vi "Simulation Trace Element.vi"(8 "error in (no error)":errorcluster, 10 "sensors":T5={"net distance (mm)"=0, "net angle (deg)"=0, "accelerometer"={"x axis (g)"=0.0, "y axis (g)"=0.0, "z axis (g)"=0.0}, "iRobot Sensors"={"Bumps + Wheel Drops"={"Wheeldrop Caster"=FALSE, "Wheeldrop Left"=FALSE, "Wheeldrop Right"=FALSE, "Bump Left"=FALSE, "Bump Right"=FALSE}, "Wall"=FALSE, "Cliff Left"=FALSE, "Cliff Front Left"=FALSE, "Cliff Front Right"=FALSE, "Cliff Right"=FALSE, "Wall Signal"=0, "Cliff Left Signal"=0, "Cliff Front Left Signal"=0, "Cliff Front Right Signal"=0, "Cliff Right Signal"=0, "Buttons"={"Advance"=FALSE, "Play"=FALSE}, "Virtual Wall"=FALSE, "# Stream Packets"=0, "Requested Velocity (mm/s)"=0, "Requested Radius (mm)"=0, "Requested Right Wheel Velocity (mm/s)"=0, "Requested Left Wheel Velocity (mm/s)"=0, "Distance (mm)"=0, "Angle (deg)"=0, "Song Playing"=FALSE, "Song Number"=0, "Charging State"=enum."Not Charging", "Voltage (mV)"=0, "Current (mA)"=0, "Battery Temperature (deg C)"=0, "Battery Charge (mAh)"=0, "Battery Capacity (mAh)"=0, "Charging Sources"={"Internal Charger"=FALSE, "Home Base"=FALSE}, "OI Mode"=enum."Off", "Digital Inputs"={"Digital Input 0"=FALSE, "Digital Input 1"=FALSE, "Digital Input 2"=FALSE, "Digital Input 3"=FALSE, "Device Detect"=FALSE}, "Drivers & Wheel Overcurrent"={"Low-Side Driver 0"=FALSE, "Low-Side Driver 1"=FALSE, "Low-Side Driver 2"=FALSE, "Left Wheel"=FALSE, "Right Wheel"=FALSE}, "Analog Signal"=0, "Infrared"=255}, "Is Simulator?"=FALSE} {"iRobot Sensors"."Infrared" format="%02x"; "accelerometer"."z axis (g)" format="%.3f"; "accelerometer"."y axis (g)" format="%.3f"; "accelerometer"."x axis (g)" format="%.3f"}, 11 "simulator":T1={"configuration"={"maxTime"=5.0, "enableVisualization"=TRUE, "statechart"=path "iRobot Navigation State Machine.vi", "environment"=path "simulation configuration.ini", "record"=path "Simulation Record.xml", "autograde?"=TRUE, "interactive?"=FALSE, "feedback mode"=enum."debug navigation"}, "Bump Sensors"=[], "Distance Sensors"=[], "Accelerometer"=refnum, "Wall Sensor"=refnum, "Statechart\ndisplay"=refnum, "Body"=refnum, "Left Motor"=refnum, "Right Motor"=refnum, "first step?"=FALSE}) -> (0 "error out":errorcluster, 2 "trace element":T4={"sensors"={"net distance (mm)"=0, "net angle (deg)"=0, "accelerometer"={"x axis (g)"=0.0, "y axis (g)"=0.0, "z axis (g)"=0.0}, "iRobot Sensors"={"Bumps + Wheel Drops"={"Wheeldrop Caster"=FALSE, "Wheeldrop Left"=FALSE, "Wheeldrop Right"=FALSE, "Bump Left"=FALSE, "Bump Right"=FALSE}, "Wall"=FALSE, "Cliff Left"=FALSE, "Cliff Front Left"=FALSE, "Cliff Front Right"=FALSE, "Cliff Right"=FALSE, "Wall Signal"=0, "Cliff Left Signal"=0, "Cliff Front Left Signal"=0, "Cliff Front Right Signal"=0, "Cliff Right Signal"=0, "Buttons"={"Advance"=FALSE, "Play"=FALSE}, "Virtual Wall"=FALSE, "# Stream Packets"=0, "Requested Velocity (mm/s)"=0, "Requested Radius (mm)"=0, "Requested Right Wheel Velocity (mm/s)"=0, "Requested Left Wheel Velocity (mm/s)"=0, "Distance (mm)"=0, "Angle (deg)"=0, "Song Playing"=FALSE, "Song Number"=0, "Charging State"=enum."Not Charging", "Voltage (mV)"=0, "Current (mA)"=0, "Battery Temperature (deg C)"=0, "Battery Charge (mAh)"=0, "Battery Capacity (mAh)"=0, "Charging Sources"={"Internal Charger"=FALSE, "Home Base"=FALSE}, "OI Mode"=enum."Off", "Digital Inputs"={"Digital Input 0"=FALSE, "Digital Input 1"=FALSE, "Digital Input 2"=FALSE, "Digital Input 3"=FALSE, "Device Detect"=FALSE}, "Drivers & Wheel Overcurrent"={"Low-Side Driver 0"=FALSE, "Low-Side Driver 1"=FALSE, "Low-Side Driver 2"=FALSE, "Left Wheel"=FALSE, "Right Wheel"=FALSE}, "Analog Signal"=0, "Infrared"=255}, "Is Simulator?"=FALSE}, "position"={"x (m)"=0.0, "y (m)"=0.0, "z (m)"=0.0}, "orientation"={"roll (deg)"=0.0, "pitch (deg)"=0.0, "yaw (deg)"=0.0}, "Simulation Time (s)"=0.0} {"sensors"."iRobot Sensors"."Infrared" format="%02x"; "sensors"."accelerometer"."z axis (g)" format="%.3f"; "sensors"."accelerometer"."y axis (g)" format="%.3f"; "sensors"."accelerometer"."x axis (g)" format="%.3f"}, 3 "simulator":T1={"configuration"={"maxTime"=5.0, "enableVisualization"=TRUE, "statechart"=path "iRobot Navigation State Machine.vi", "environment"=path "simulation configuration.ini", "record"=path "Simulation Record.xml", "autograde?"=TRUE, "interactive?"=FALSE, "feedback mode"=enum."debug navigation"}, "Bump Sensors"=[], "Distance Sensors"=[], "Accelerometer"=refnum, "Wall Sensor"=refnum, "Statechart\ndisplay"=refnum, "Body"=refnum, "Left Motor"=refnum, "Right Motor"=refnum, "first step?"=FALSE})   [LabVIEW 2013]
doc: "Reads parameters from the simulator sensors and packages them into a single trace element."
uses:
  shared/Sensors.ctl
  iRobot/Sensor/Accelerometer.ctl
  iRobot/Sensor/Sensor Group 6.ctl
  iRobot/Sensor/Bumps + Wheel Drops.ctl
  iRobot/Sensor/Buttons.ctl
  iRobot/Sensor/Charging State.ctl
  iRobot/Sensor/Charging Sources Available.ctl
  iRobot/Sensor/OI Mode.ctl
  iRobot/Sensor/Cargo Bay Digital Inputs.ctl
  iRobot/Sensor/Low-Side Driver + Wheel Overcurrent.ctl
  Simulation Trace Element.ctl
  Simulated iRobot Position.ctl
  Simulated iRobot Orientation.ctl
  Simulator.ctl
  <instrlib>/DC Motor Controller/HAIOL/DC Motor Controller.lvclass
  CyberSim interface/Simulation Configuration.ctl
  autograder/feedbackMode.ctl
  <vilib>/robotics/Simulator/Interface/Simulator References/Get World Reference.vi
  <resource>/objmgr/LVODE.rc
  <vilib>/robotics/Simulator/NI_Robotics_Simulator.lvlib
  <vilib>/robotics/Kinematics/NI_Kinematics.lvlib
panel:
  # "Electrical: charging, battery, OI mode"
  # "Sensors: bump, cliff, button, wheel drop, wall, virtual wall"
  # "Motion: distance, angle, requested velocity"
  # "Cargo Bay: I/O, overcurrent, infrared"
  # "Song"
  # "Electrical: charging, battery, OI mode"
  # "Sensors: bump, cliff, button, wheel drop, wall, virtual wall"
  # "Motion: distance, angle, requested velocity"
  # "Cargo Bay: I/O, overcurrent, infrared"
  # "Song"
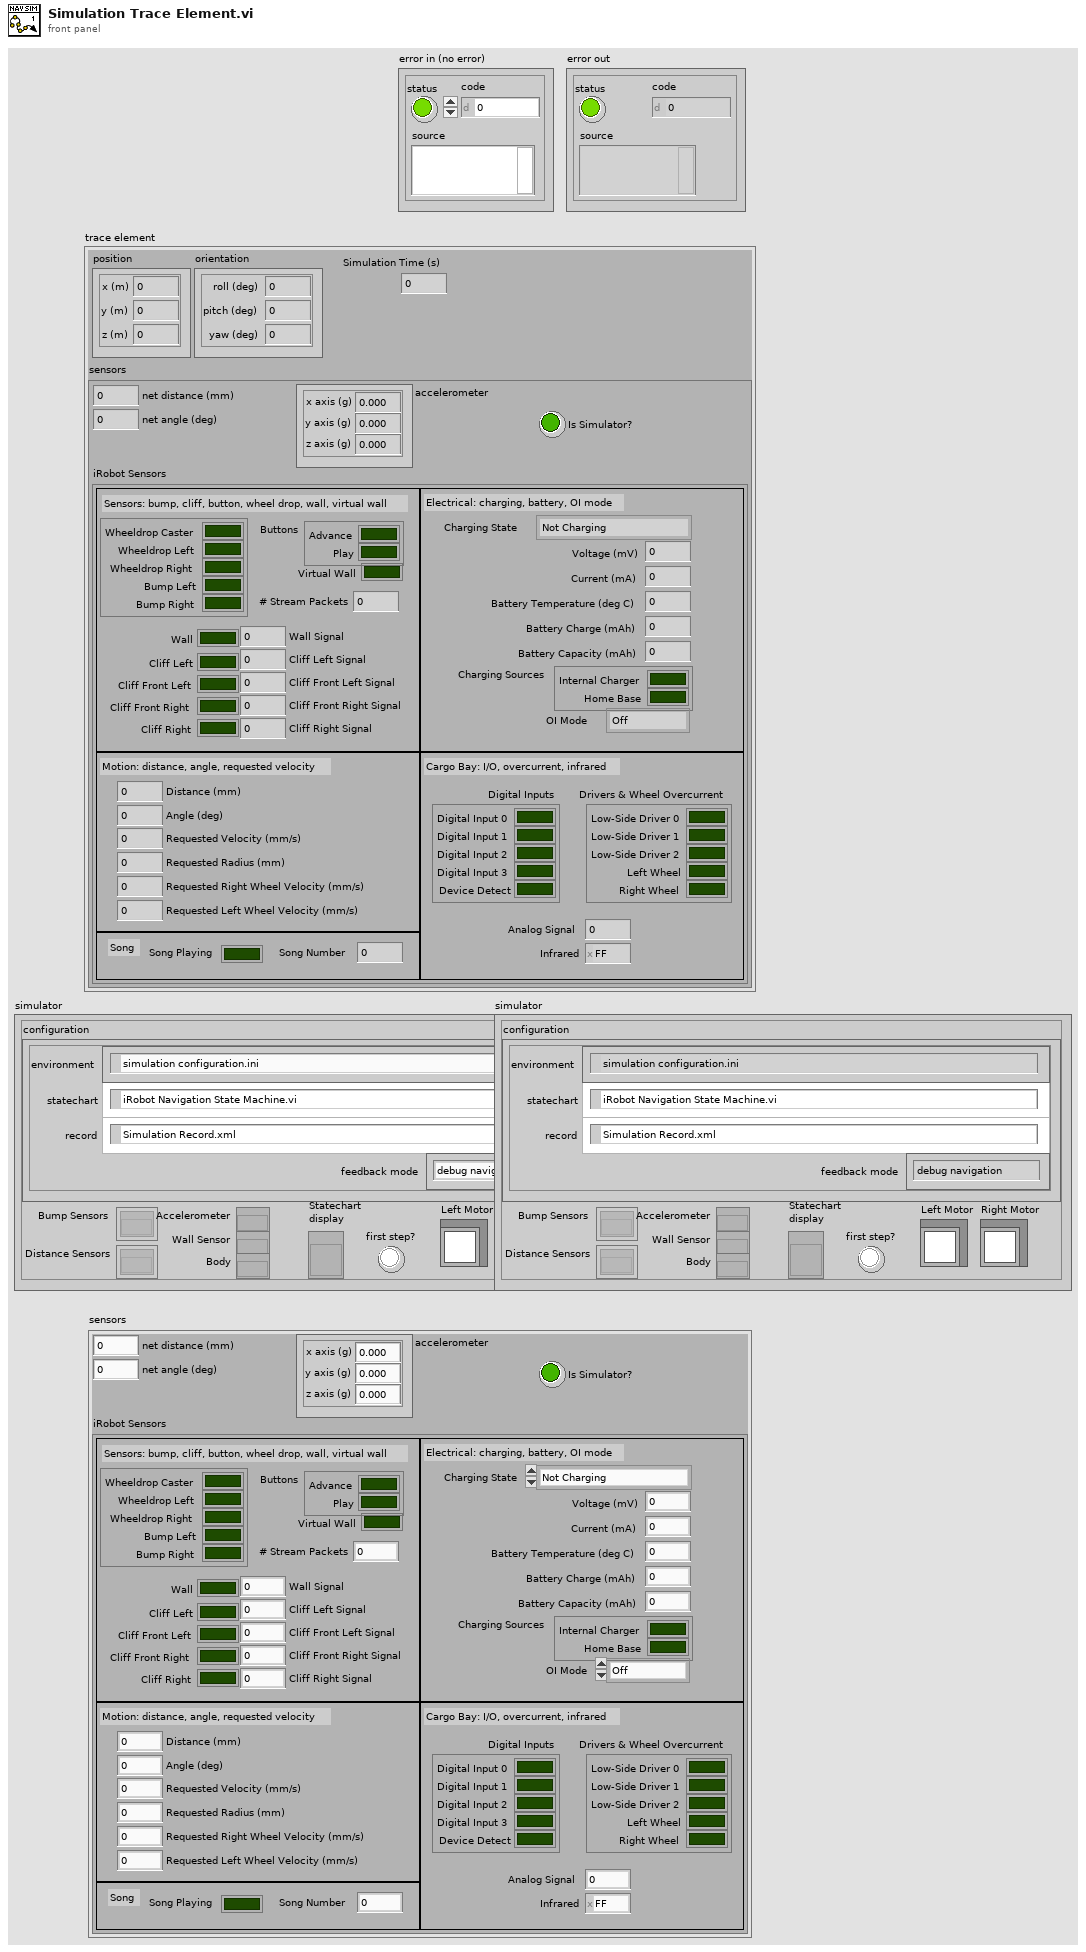
[diagram p1: front panel]
types:
  T1 = typedef "Simulator.ctl" = cluster{"configuration":T2, "Bump Sensors":refnum<k20>[], "Distance Sensors":refnum<k20>[], "Accelerometer":refnum<k20>, "Wall Sensor":refnum<k20>, "Statechart\ndisplay":refnum<vi>, "Body":refnum<k20>, "Left Motor":refnum<class "DC Motor Controller.lvclass">, "Right Motor":refnum<class "DC Motor Controller.lvclass">, "first step?":bool}
  T2 = typedef "Simulation Configuration.ctl" = cluster{"maxTime":sgl, "enableVisualization":bool, "statechart":path, "environment":path, "record":path, "autograde?":bool, "interactive?":bool, "feedback mode":T3}
  T3 = typedef "feedbackMode.ctl" = enum32{"debug navigation", "debug hill climb", "autograde navigation", "autograde hill climb"}
  T4 = typedef "Simulation Trace Element.ctl" = cluster{"sensors":T5, "position":T15, "orientation":T16, "Simulation Time (s)":sgl}
  T5 = typedef "Sensors.ctl" = cluster{"net distance (mm)":i32, "net angle (deg)":i32, "accelerometer":T6, "iRobot Sensors":T7, "Is Simulator?":bool}
  T6 = typedef "Accelerometer.ctl" = cluster{"x axis (g)":dbl, "y axis (g)":dbl, "z axis (g)":dbl}
  T7 = typedef "Sensor Group 6.ctl" = cluster{"Bumps + Wheel Drops":T8, "Wall":bool, "Cliff Left":bool, "Cliff Front Left":bool, "Cliff Front Right":bool, "Cliff Right":bool, "Wall Signal":u16, "Cliff Left Signal":u16, "Cliff Front Left Signal":u16, "Cliff Front Right Signal":u16, "Cliff Right Signal":u16, "Buttons":T9, "Virtual Wall":bool, "# Stream Packets":u8, "Requested Velocity (mm/s)":i16, "Requested Radius (mm)":i16, "Requested Right Wheel Velocity (mm/s)":i16, "Requested Left Wheel Velocity (mm/s)":i16, "Distance (mm)":i32, "Angle (deg)":i32, "Song Playing":bool, "Song Number":u8, "Charging State":T10, "Voltage (mV)":u16, "Current (mA)":i16, "Battery Temperature (deg C)":i8, "Battery Charge (mAh)":u16, "Battery Capacity (mAh)":u16, "Charging Sources":T11, "OI Mode":T12, "Digital Inputs":T13, "Drivers & Wheel Overcurrent":T14, "Analog Signal":u16, "Infrared":u8}
  T8 = typedef "Bumps + Wheel Drops.ctl" = cluster{"Wheeldrop Caster":bool, "Wheeldrop Left":bool, "Wheeldrop Right":bool, "Bump Left":bool, "Bump Right":bool}
  T9 = typedef "Buttons.ctl" = cluster{"Advance":bool, "Play":bool}
  T10 = typedef "Charging State.ctl" = enum16{"Not Charging", "Reconditioning Charging", "Full Charging", "Trickle Charging", "Waiting", "Charging Fault Condition"}
  T11 = typedef "Charging Sources Available.ctl" = cluster{"Internal Charger":bool, "Home Base":bool}
  T12 = typedef "OI Mode.ctl" = enum16{"Off", "Passive", "Safe", "Full"}
  T13 = typedef "Cargo Bay Digital Inputs.ctl" = cluster{"Digital Input 0":bool, "Digital Input 1":bool, "Digital Input 2":bool, "Digital Input 3":bool, "Device Detect":bool}
  T14 = typedef "Low-Side Driver + Wheel Overcurrent.ctl" = cluster{"Low-Side Driver 0":bool, "Low-Side Driver 1":bool, "Low-Side Driver 2":bool, "Left Wheel":bool, "Right Wheel":bool}
  T15 = typedef "Simulated iRobot Position.ctl" = cluster{"x (m)":sgl, "y (m)":sgl, "z (m)":sgl}
  T16 = typedef "Simulated iRobot Orientation.ctl" = cluster{"roll (deg)":sgl, "pitch (deg)":sgl, "yaw (deg)":sgl}
  T17 = cluster{"Position[0]":sgl, "Position[1]":sgl, "Position[2]":sgl}
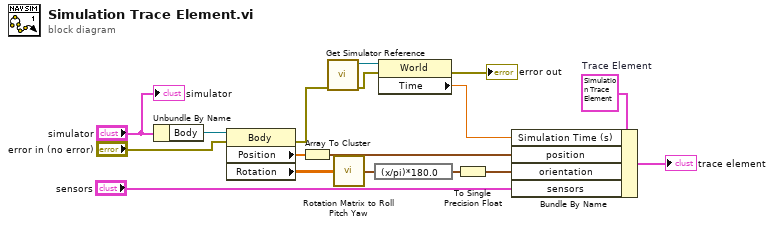
[diagram p0: block diagram]
diagram:
  w16 = T4 {"sensors"={"net distance (mm)"=0, "net angle (deg)"=0, "accelerometer"={"x axis (g)"=0.0, "y axis (g)"=0.0, "z axis (g)"=0.0}, "iRobot Sensors"={"Bumps + Wheel Drops"={"Wheeldrop Caster"=FALSE, "Wheeldrop Left"=FALSE, "Wheeldrop Right"=FALSE, "Bump Left"=FALSE, "Bump Right"=FALSE}, "Wall"=FALSE, "Cliff Left"=FALSE, "Cliff Front Left"=FALSE, "Cliff Front Right"=FALSE, "Cliff Right"=FALSE, "Wall Signal"=0, "Cliff Left Signal"=0, "Cliff Front Left Signal"=0, "Cliff Front Right Signal"=0, "Cliff Right Signal"=0, "Buttons"={"Advance"=FALSE, "Play"=FALSE}, "Virtual Wall"=FALSE, "# Stream Packets"=0, "Requested Velocity (mm/s)"=0, "Requested Radius (mm)"=0, "Requested Right Wheel Velocity (mm/s)"=0, "Requested Left Wheel Velocity (mm/s)"=0, "Distance (mm)"=0, "Angle (deg)"=0, "Song Playing"=FALSE, "Song Number"=0, "Charging State"=enum."Not Charging", "Voltage (mV)"=0, "Current (mA)"=0, "Battery Temperature (deg C)"=0, "Battery Charge (mAh)"=0, "Battery Capacity (mAh)"=0, "Charging Sources"={"Internal Charger"=FALSE, "Home Base"=FALSE}, "OI Mode"=enum."Off", "Digital Inputs"={"Digital Input 0"=FALSE, "Digital Input 1"=FALSE, "Digital Input 2"=FALSE, "Digital Input 3"=FALSE, "Device Detect"=FALSE}, "Drivers & Wheel Overcurrent"={"Low-Side Driver 0"=FALSE, "Low-Side Driver 1"=FALSE, "Low-Side Driver 2"=FALSE, "Left Wheel"=FALSE, "Right Wheel"=FALSE}, "Analog Signal"=0, "Infrared"=0}, "Is Simulator?"=FALSE}, "position"={"x (m)"=0.0, "y (m)"=0.0, "z (m)"=0.0}, "orientation"={"roll (deg)"=0.0, "pitch (deg)"=0.0, "yaw (deg)"=0.0}, "Simulation Time (s)"=0.0}  # Trace Element
  n1 = Unbundle By Name("simulator") -> ("Body"=w17:refnum<k20>)
  n2 = property class="Body"(reference=w17, error in="error in (no error)") -> (error out=w13:errorcluster, "Position"=w7:sgl[], "Rotation"=w2:sgl[][])  [unwired: 1 out]
  n3 = Array To Cluster(array=w7) -> (cluster=w6:T17)
  n4 = call-poly <vilib>:"Get Simulator Reference.vi"("error in (no error)"=w13) -> ("error out"=w14:errorcluster, "world ref"=w15:refnum<k20>)  [unwired: 9 in]
  n5 = call <vilib>:"Rotation Matrix to Roll Pitch Yaw.vi"("rotation matrix"=w2) -> ("angles"=w5:cluster{"roll":dbl, "pitch":dbl, "yaw":dbl})
  n6 = expression code="(x/pi)*180.0" ("radians to degrees")(w5) -> (w4:cluster{"roll":dbl, "pitch":dbl, "yaw":dbl})
  n7 = property class="World"(reference=w15, error in=w14) -> (error out=→"error out":errorcluster, "Time"=w8:sgl)  [unwired: 1 out]
  n8 = To Single Precision Float(number=w4) -> (single precision float=w3:cluster{"roll":sgl, "pitch":sgl, "yaw":sgl})
  n9 = Bundle By Name(cluster=w16, "Simulation Time (s)"=w8, "position"=w6, "orientation"=w3, "sensors"="sensors") -> (→"trace element":T4)
  "simulator" <- "simulator"
